vi "Test Instruments.vi"(0 "Instrument List In":T1[](array[typedef]) {"Private"."Offset" format="%^_3e"; "Private"."Scale Factors" format="%^_3e"}) -> (1 "Instrument List Out":T1[](array[typedef]) {"Private"."Offset" format="%^_3e"; "Private"."Scale Factors" format="%^_3e"}, 2 "Test Data":dbl[](array[numeric]) format="%_6e")   [LabVIEW 2025]
doc: "Author: Scott Hannahs <sth@magnet.fsu.edu>\n\nThis software is licensed for use under the “MIT License\"\nCopyright (c) 2025 Scott Hannahs, sth@sth@magnet.sthnet.net\n\nPermission is hereby granted, free of charge, to any person obtaining a copy of this software and associated documentation files (the \"Software\"), to deal in the Software without restriction, including without limitation the rights to use, copy, modify, merge, publish, distribute, sublicense, and/or sell copies of the Software, and to permit persons to whom the Software is furnished to do so, subject to the following conditions: The above copyright notice and this permission notice shall be included in all copies or substantial portions of the Software.\n\nTHE SOFTWARE IS PROVIDED \"AS IS\", WITHOUT WARRANTY OF ANY KIND, EXPRESS OR IMPLIED, INCLUDING BUT NOT LIMITED TO THE WARRANTIES OF MERCHANTABILITY, FITNESS FOR A PARTICULAR PURPOSE AND NONINFRINGEMENT. IN NO EVENT SHALL THE AUTHORS OR COPYRIGHT HOLDERS BE LIABLE FOR ANY CLAIM, DAMAGES OR OTHER LIABILITY, WHETHER IN AN ACTION OF CONTRACT, TORT OR OTHERWISE, ARISING FROM, OUT OF OR IN CONNECTION WITH THE SOFTWARE OR THE USE OR OTHER DEALINGS IN THE SOFTWARE."
uses:
  Sub Controls/Instrument Properties.ctl
  Sub Controls/Public.ctl
  Sub Controls/Private.ctl
  Sub Controls/Instrument Ref.ctl
  Sub Controls/SystemCheckBox-resize.ctl
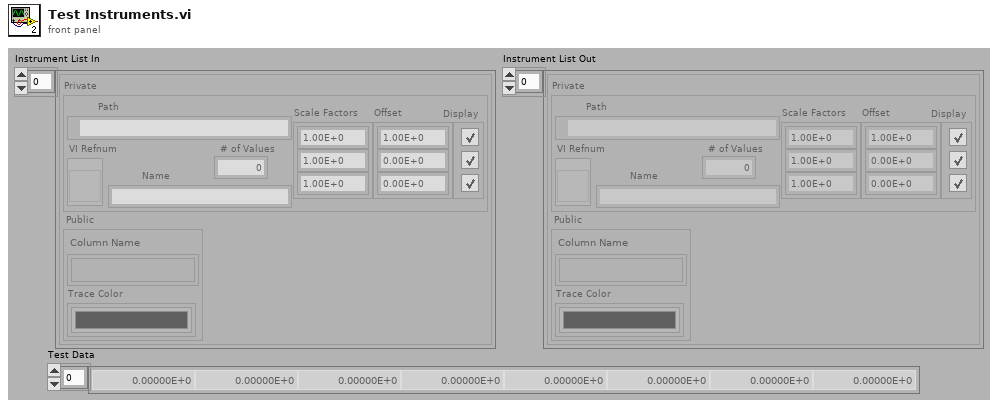
[diagram p1: front panel]
types:
  T1 = typedef "Instrument Properties.ctl" = cluster{"Public":T2, "Private":T3}
  T2 = typedef "Public.ctl" = cluster{"Column Name":string[], "Trace Color":u32[]}
  T3 = typedef "Private.ctl" = cluster{"Path":path, "VI Refnum":T4, "Name":string, "# of Values":i32, "Scale Factors":dbl[], "Display":T5[], "Offset":dbl[]}
  T4 = typedef "Instrument Ref.ctl" = refnum<vi>
  T5 = typedef "SystemCheckBox-resize.ctl" = bool
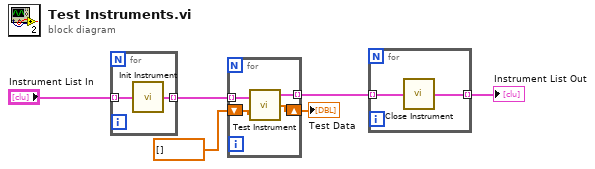
[diagram p0: block diagram]
diagram:
  n1 = for {
    tunnel: "Instrument List In" -> [w8] mode=indexing
    tunnel: [w7] -> w3 mode=indexing
    n2 = call "Init Instrument.vi"("Instrument Prop"=w8) -> ("Instrument Prop 2"=w7:T1)
  }
  n3 = for {
    tunnel: w3 -> [w12] mode=indexing
    tunnel: [w10] -> w5 mode=indexing
    shift-right: [w9] -> w2
    shift-left: dbl[] [] ("Array 2") -> [w11]
    n4 = call "Test Instrument.vi"("Instrument Prop In"=w12, "Array"=w11) -> ("Instrument Prop Out"=w10:T1, "Array 2"=w9:dbl[])  [unwired: 1 out]
  }
  "Test Data" <- w2
  n5 = for {
    tunnel: w5 -> [w14] mode=indexing
    tunnel: [w13] -> w6 mode=indexing
    n6 = call "Close Instrument.vi"("Instrument Prop"=w14) -> ("Instrument Prop 2"=w13:T1)
  }
  "Instrument List Out" <- w6
